vi "Close.vi"(8 "error in (no error)":errorcluster, 11 "PwrMtr_U2k in":refnum<class "PwrMtr_U2k.lvclass">) -> (0 "error out":errorcluster)   [LabVIEW 2014, in "PwrMtr_U2k.lvclass"]
uses:
  PwrMtr_U2k.lvclass
  PwrMtr_U2k.lvclass/PwrMtr_U2k.ctl
  data/Agilent U2000 Series.lvlib
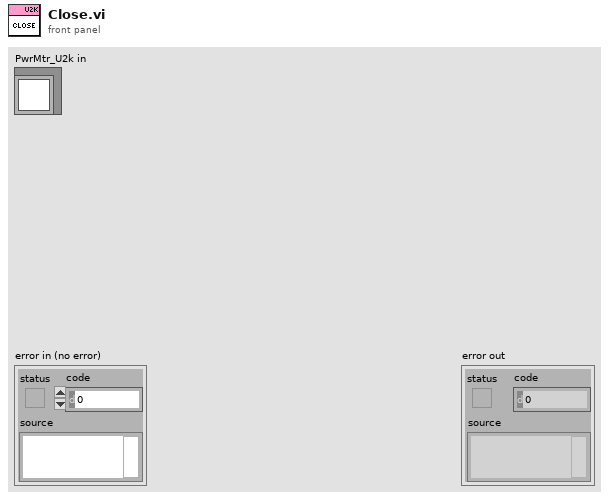
[diagram p1: front panel]
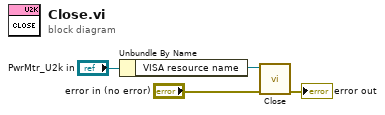
[diagram p0: block diagram]
diagram:
  n1 = Unbundle By Name("PwrMtr_U2k in") -> ("VISA resource name"=w2:refnum<visa-resource-name>)
  n2 = call "Close.vi"("error in (no error)"="error in (no error)", "VISA resource name"=w2) -> ("error out"=→"error out":errorcluster)  [unwired: 9 out]
